vi "add_CameraSettings.vi"(4 "Camera Settings":T1={"FPS"=20.0, "Camera Controls"=[], "Width"=0, "Height"=0}, 5 "msg in":string) -> (2 "msg out":string)   [LabVIEW 2012]
uses:
  <userlib>/ROSforLV/ROS/MessageBuilding/std_msgs/subs/i32Scalar.vi
  <userlib>/ROSforLV/ROS/MessageBuilding/std_msgs/subs/float32Scalar.vi
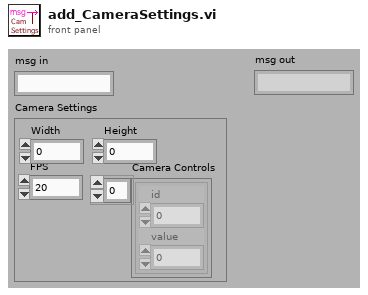
[diagram p1: front panel]
types:
  T1 = cluster{"FPS":sgl, "Camera Controls":cluster{"id":i32, "value":i32}[], "Width":i32, "Height":i32}
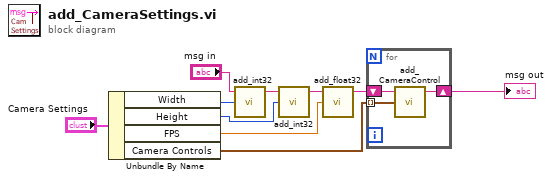
[diagram p0: block diagram]
diagram:
  n1 = Unbundle By Name("Camera Settings") -> ("Width"=w9:i32, "Height"=w8:i32, "FPS"=w5:sgl, "Camera Controls"=w3:cluster{"id":i32, "value":i32}[])
  n2 = call-poly <userlib>:"add_int32.vi"("Numeric"=w9, "msg in"="msg in") -> ("msg out"=w7:string)  [unwired: 3 in]
  n3 = call-poly <userlib>:"add_int32.vi"("Numeric"=w8, "msg in"=w7) -> ("msg out"=w6:string)  [unwired: 3 in]
  n4 = call-poly <userlib>:"add_float32.vi"("Numeric"=w5, "msg in"=w6) -> ("msg out"=w4:string)  [unwired: 3 in]
  n5 = for {
    shift-right: [w12] -> w1
    shift-left: w4 -> [w13]
    tunnel: w3 -> [w11] mode=indexing
    n6 = call <userlib>:"add_CameraControl.vi"("Camera Control"=w11, "msg in"=w13) -> ("msg out"=w12:string)  [unwired: 3 in]
  }
  "msg out" <- w1
